vi "Check and Create Folder.vi"(11 "appended path":path) -> (3 "dup path":path)   [LabVIEW 2013]
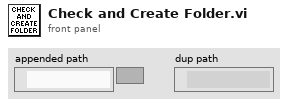
[diagram p1: front panel]
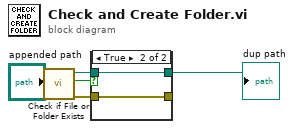
[diagram p0: block diagram]
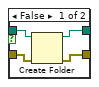
[diagram p2: hidden frame]
diagram:
  n1 = call <vilib>:"Check if File or Folder Exists.vi"("path"="appended path") -> ("error out"=w3:errorcluster, "file or folder exists?"=w1:bool, "dup path"=w2:path)  [unwired: 8 in]
  n2 = case shown="True" w1 {
    tunnel: w2 -> [w8 w11]
    tunnel: [w7 w11] -> w5
    tunnel: w3 -> [w9 w10]
    tunnel: [w6 w10] -> _
    frame False {
      n3 = Create Folder(path (use dialog)=w8, error in=w9) -> (created path=w7:path, error out=w6:errorcluster)  [unwired: 1 in, 1 out]
    }
    frame True {
    }
  }
  "dup path" <- w5
